vi "Dequeue Blocking Callbacks.vi"(8 "error in (no error)":errorcluster, 11 "Future in":refnum<class "Future.lvclass">) -> (0 "error out":errorcluster, 2 "Sync Callbacks":refnum<class "Blocking Callback.lvclass">[](array[class]), 3 "Future out":refnum<class "Future.lvclass">)   [LabVIEW 2017, in "Promise Future.lvlib" / "Future.lvclass"]
uses:
  Future.lvclass
  Callback/Blocking Callback.lvclass
  Future.lvclass/Future.ctl
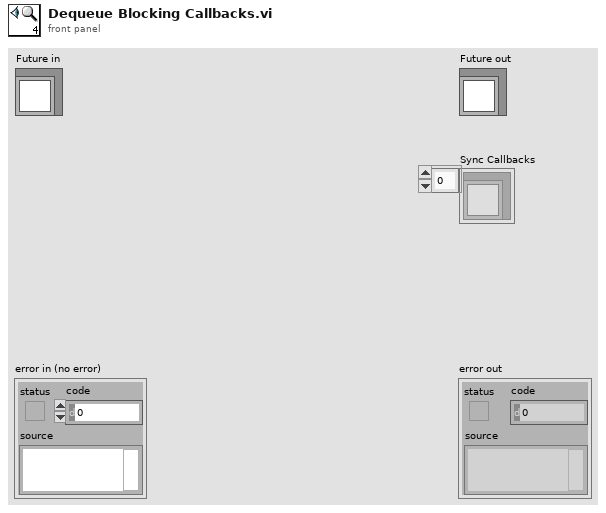
[diagram p1: front panel]
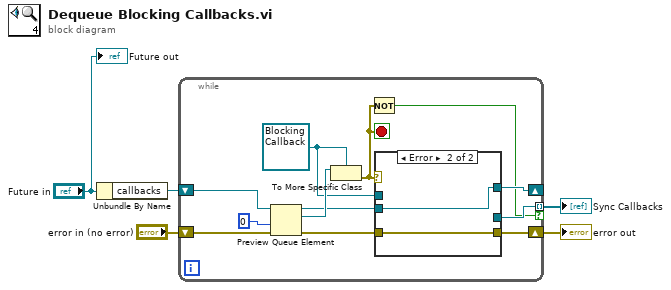
[diagram p0: block diagram]
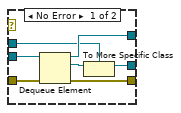
[diagram p2: hidden frame]
diagram:
  n1 = Unbundle By Name("Future in") -> ("callbacks"=w2:refnum<queue>)
  n2 = while {
    shift-right: [w9] -> w4
    shift-left: "error in (no error)" -> [w13]
    shift-right: [w12] -> _
    shift-left: w2 -> [w17]
    tunnel: [w11] -> w1 mode=indexing if=w10
    stop <- w6 stop-if-true
    w7 = refnum<class "Blocking Callback.lvclass"> refnum ("Promise Future.lvlib:Synchronous Callback.lvclass")
    n3 = Preview Queue Element(queue=w17, timeout in ms (-1)=0, error in (no error)=w13) -> (queue out=w15:refnum<queue>, element=w16:refnum<class "Callback.lvclass">, error out=w14:errorcluster)  [unwired: 1 out]
    n4 = To More Specific Class(target class=w7, reference=w16) -> (error out=w6:errorcluster)  [unwired: 1 in, 1 out]
    n5 = Not(x=w6) -> (.not. x?=w10:bool)
    n6 = case shown="Error" w6 {
      tunnel: w15 -> [w24 w26]
      tunnel: w14 -> [w23 w25]
      tunnel: [w22 w25] -> w9
      tunnel: [w21 w26] -> w12
      tunnel: [w19 _] -> w11
      tunnel: w7 -> [w18 _]
      frame No Error {
        n7 = Dequeue Element(queue=w24, error in (no error)=w23) -> (queue out=w21:refnum<queue>, element=w20:refnum<class "Callback.lvclass">, error out=w22:errorcluster)  [unwired: 1 in, 1 out]
        n8 = To More Specific Class(target class=w18, reference=w20) -> (specific class reference=w19:refnum<class "Blocking Callback.lvclass">)  [unwired: 1 in, 1 out]
      }
      frame Error {
      }
    }
  }
  "error out" <- w4
  "Sync Callbacks" <- w1
  "Future out" <- "Future in"
